vi "Initialize.vi"(4 "Password":string, 6 "Username":string, 7 "connection information":string, 8 "error in (no error)":errorcluster, 9 "columns":string[](array[string]), 10 "table":string, 11 "DbMeasurement in":refnum<class "DbMeasurement.lvclass">) -> (0 "error out":errorcluster, 3 "DbMeasurement out":refnum<class "DbMeasurement.lvclass">)   [LabVIEW 2013, in "DbMeasurement.lvclass"]
doc: "This public method initializes the measurement class, obtaining a data queue and opening the database file."
uses:
  DbMeasurement.lvclass
  DbMeasurement.lvclass/DbMeasurement.ctl
  BaseMeasurement/BaseMeasurement.lvclass/BaseMeasurement.ctl
  BaseMeasurement/BaseMeasurement.lvclass
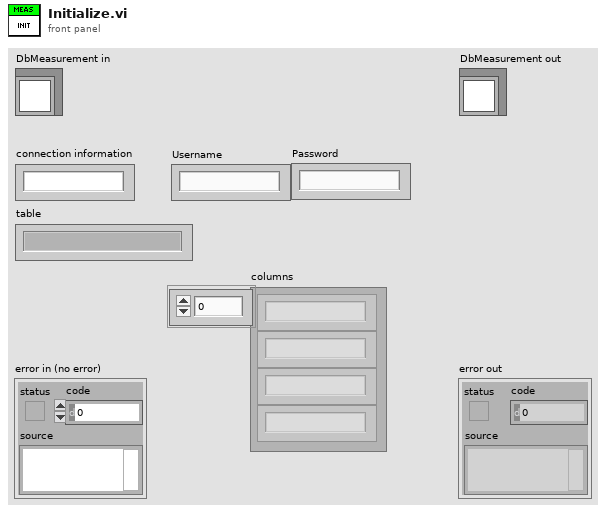
[diagram p1: front panel]
types:
  T1 = cluster{dbl, "JSON string":string, "JSON string":string, i16, "date/time string":string, dbl, "JSON string":string, "JSON string":string}
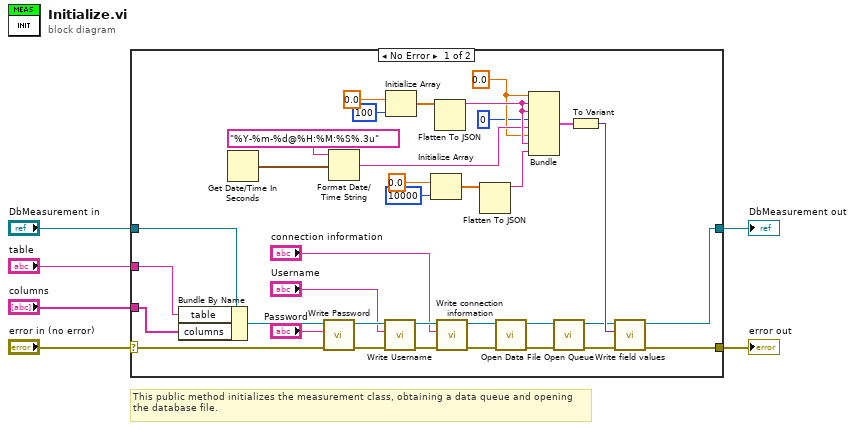
[diagram p0: block diagram]
diagram:
  # "This public method initializes the measurement class, obtaining a data queue and opening the database file."
  n1 = case shown="No Error" "error in (no error)" {
    selector: "error in (no error)" -> [w29 w43]
    tunnel: [w10 w43] -> w5
    tunnel: [w7 w42] -> w3
    tunnel: "DbMeasurement in" -> [w37 w42]
    tunnel: "table" -> [w36 _]
    tunnel: "columns" -> [w35 _]
    frame No Error {
      w21 = 0.0
      n2 = Bundle By Name(cluster=w37, "table"=w36, "columns"=w35) -> (w32:refnum<class "DbMeasurement.lvclass">)
      n3 = Get Date/Time In Seconds() -> (seconds since 1Jan1904=w16:timestamp)
      n4 = call "Write Password.vi"("error in (no error)"=w29, "Password"="Password", "BaseMeasurement in"=w32) -> ("error out"=w34:errorcluster, "BaseMeasurement out"=w31:refnum<class "DbMeasurement.lvclass">)  [unwired: 7 in]
      n5 = Format Date/Time String(time format string (%c)="%Y-%m-%d@%H:%M:%S%.3u", seconds (now)=w16) -> (date/time string=w22:string)  [unwired: 1 in]
      n6 = call "Write Username.vi"("error in (no error)"=w34, "Username"="Username", "BaseMeasurement in"=w31) -> ("error out"=w33:errorcluster, "BaseMeasurement out"=w30:refnum<class "DbMeasurement.lvclass">)  [unwired: 7 in]
      n7 = Initialize Array(0.0 ("element"), 100 ("dimension size")) -> (w14:dbl[])
      n8 = Initialize Array(0.0 ("element"), 10000 ("dimension size")) -> (w17:dbl[])
      n9 = Flatten To JSON(anything=w14) -> (JSON string=w23:string)  [unwired: 2 in, 1 out]
      n10 = call "Write connection information.vi"("error in (no error)"=w33, "connection information"="connection information", "BaseMeasurement in"=w30) -> ("error out"=w41:errorcluster, "BaseMeasurement out"=w40:refnum<class "DbMeasurement.lvclass">)  [unwired: 7 in]
      n11 = Flatten To JSON(anything=w17) -> (JSON string=w24:string)  [unwired: 2 in, 1 out]
      n12 = call "Open Data File.vi"("error in (no error)"=w41, "DbMeasurement in"=w40) -> ("error out"=w39:errorcluster, "DbMeasurement out"=w38:refnum<class "DbMeasurement.lvclass">)  [unwired: 8 in]
      n13 = Bundle(w21, "JSON string"=w23, "JSON string"=w23, i16 0, "date/time string"=w22, w21, "JSON string"=w23, "JSON string"=w24) -> (w25:T1)  [unwired: 1 in]
      n14 = call "Open Queue.vi"("error in (no error)"=w39, "DbMeasurement in"=w38) -> ("error out"=w11:errorcluster, "DbMeasurement out"=w8:refnum<class "DbMeasurement.lvclass">)  [unwired: 8 in]
      n15 = To Variant(anything=w25) -> (Variant=w9:variant)
      n16 = call "Write field values.vi"("error in (no error)"=w11, "field values"=w9, "DbMeasurement in"=w8) -> ("error out"=w10:errorcluster, "DbMeasurement out"=w7:refnum<class "DbMeasurement.lvclass">)  [unwired: 7 in]
    }
    frame Error {
    }
  }
  "error out" <- w5
  "DbMeasurement out" <- w3
